vi "DecodeXceiverRev.vi"(7 "error in":errorcluster, 10 "Byte Array In":u8[](array[numeric]) format="%x") -> (0 "error out":errorcluster, 2 "Valid Rev?":bool, 3 "Rev String Out":string)   [LabVIEW 2015]
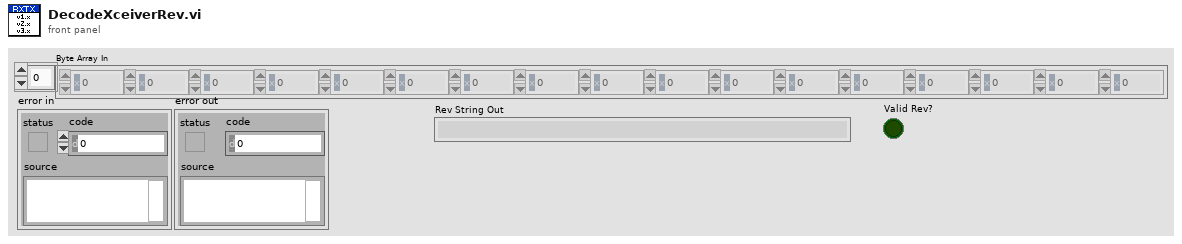
[diagram p1: front panel]
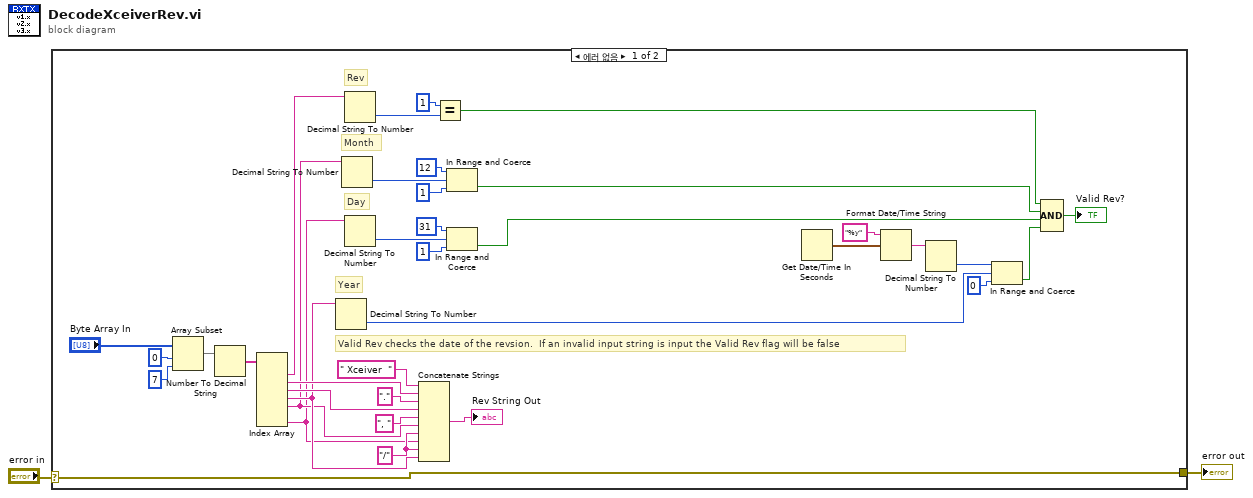
[diagram p0: block diagram]
diagram:
  n1 = case shown="에러 없음" "error in" {
    selector: "error in" -> [w3 w39]
    tunnel: [w3 w39] -> w1
    frame No Error {
      w30 = "/" ("string")
      # "Year"
      # "Day"
      # "Month"
      # "Rev"
      # "Valid Rev checks the date of the revsion.  If an invalid input string is input the Valid Rev flag will be false"
      n2 = Array Subset(array="Byte Array In", index=0, length=7) -> (w37:u8[])
      n3 = Number To Decimal String(number=w37) -> (decimal integer string=w35:string[])  [unwired: 1 in]
      n4 = Index Array(array=w35) -> (element #1=w5:string, element #2=w15:string, element #3=w34:string, element #4=w14:string, element #5=w13:string, element #7=w12:string)  [unwired: 7 in, 1 out]
      n5 = Decimal String To Number(string=w14) -> (number=w23:i32)  [unwired: 2 in, 1 out]
      n6 = Decimal String To Number(string=w13) -> (number=w25:i32)  [unwired: 2 in, 1 out]
      n7 = Decimal String To Number(string=w5) -> (number=w27:i32)  [unwired: 2 in, 1 out]
      n8 = Decimal String To Number(string=w12) -> (number=w24:i32)  [unwired: 2 in, 1 out]
      n9 = Concatenate Strings(" Xceiver  " ("string"), w15, "." ("string"), w34, ", " ("string"), w13, w30, w12, w30, w14) -> (→"Rev String Out":string)
      n10 = Equal?(x=1, y=w27) -> (x = y?=w19:bool)
      n11 = In Range and Coerce(upper limit=12 ("lower limit"), x=w25, lower limit=1 ("upper limit")) -> (In Range?=w18:bool)  [unwired: 1 out]
      n12 = In Range and Coerce(upper limit=31 ("lower limit"), x=w24, lower limit=1 ("upper limit")) -> (In Range?=w17:bool)  [unwired: 1 out]
      n13 = Get Date/Time In Seconds() -> (seconds since 1Jan1904=w21:timestamp)
      n14 = Format Date/Time String(time format string (%c)="%y", seconds (now)=w21) -> (date/time string=w20:string)  [unwired: 1 in]
      n15 = Decimal String To Number(string=w20) -> (number=w10:i32)  [unwired: 2 in, 1 out]
      n16 = In Range and Coerce(upper limit=w10, x=w23, lower limit=0 ("upper limit")) -> (In Range?=w16:bool)  [unwired: 1 out]
      n17 = Compound Arithmetic op=AND(w19, w18, w17, w16) -> (→"Valid Rev?":bool)
    }
    frame Error {
    }
  }
  "error out" <- w1
